vi "DMM Measurement.vi"() -> ()   [LabVIEW 2021]
doc: "This example acquires a single measurement from a National Instruments DMM. Select the measurement function and range. Specify the resolution in digits of precision. The measured value will be displayed in the Measurement indicator. The Boolean indicator will indicate if the measured value is out of range."
uses:
  <instrlib>/niDMM/nidmm.llb/niDMM Configure Measurement Digits.vi
  <instrlib>/niDMM/nidmm.llb/niDMM Function.ctl
  <instrlib>/niDMM/nidmm.llb/niDMM Resolution in Digits.ctl
panel:
  out "error out":errorcluster
  in  "error in":errorcluster caption="error in (no error)"
  in  "Resolution in Digits":T1=5.5 items=["3 1/2"=3.5, "4 1/2"=4.5, "5 1/2"=5.5, "6 1/2"=6.5, "7 1/2"=7.5]
  out "Absolute Resolution":dbl format="%#_3p"
  in  "Measurement Type":T2
  out "Signal Out of Range":bool
  in  "Range":dbl=10.0 format="%.2f"
  in  "Device Name":refnum<k15>="Dev1"
  out "Measurement":dbl format="%.6p"
  # "For instructions select File >> VI Properties >> Documentation"
  # "Configuration"
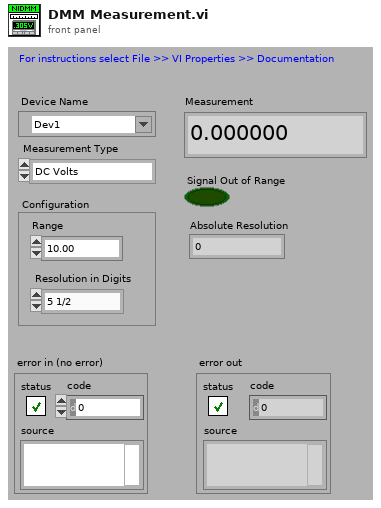
[diagram p1: front panel]
types:
  T1 = typedef "niDMM Resolution in Digits.ctl" = dbl
  T2 = typedef "niDMM Function.ctl" = enum16{"DC Volts", "AC Volts", "DC Current", "AC Current", "2-wire Resistance", "4-wire Resistance", "Diode", "Frequency", "Period", "AC Volts DC Coupled", "Capacitance", "Inductance", "Temperature"}
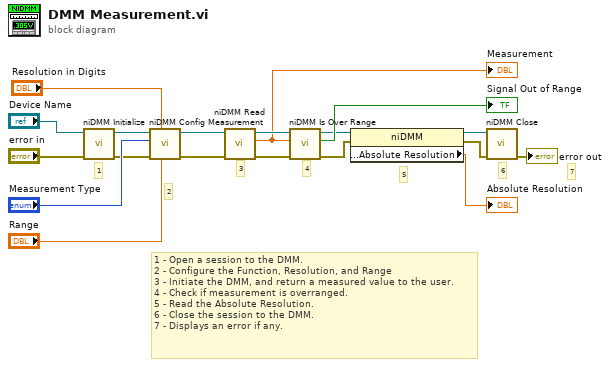
[diagram p0: block diagram]
diagram:
  # "2"
  # "1 - Open a session to the DMM.\n2 - Configure the Function, Resolution, and Range\n3 - Initiate the DMM, and return a measured value to the user.\n4 - Check if measurement is overranged.\n5 - Read the Absolute Resolution.\n6 - Close the session to the DMM.\n7 - Displays an error if any."
  # "1"
  # "7"
  # "6"
  # "5"
  # "4"
  # "3"
  n1 = call <instrlib>:"niDMM Initialize.vi"("error in (no error)"="error in", "Instrument Descriptor"="Device Name") -> ("error out"=w10:errorcluster, "instrument handle out"=w9:refnum<k15>)  [unwired: 8 in]
  n2 = call-poly <instrlib>:"niDMM Config Measurement.vi"("Range"="Range", "Resolution in Digits"="Resolution in Digits", "error in (no error)"=w10, "Function"="Measurement Type", "instrument handle"=w9) -> ("error out"=w17:errorcluster, "instrument handle out"=w16:refnum<k15>)  [unwired: 5 in]
  n3 = call <instrlib>:"niDMM Read.vi"("error in (no error)"=w17, "instrument handle"=w16) -> ("error out"=w14:errorcluster, "Measurement"=w12:dbl, "instrument handle out"=w15:refnum<k15>)  [unwired: 7 in]
  "Measurement" <- w12
  n4 = call <instrlib>:"niDMM Is Over Range.vi"("error in (no error)"=w14, "Measurement"=w12, "instrument handle"=w15) -> ("error out"=w6:errorcluster, "Over Range?"=→"Signal Out of Range":bool, "instrument handle out"=w8:refnum<k15>)  [unwired: 6 in]
  n5 = property class="niDMM"(reference=w8, error in=w6) -> (reference out=w7:refnum<k15>, error out=w5:errorcluster, "Configuration:Absolute Resolution"=→"Absolute Resolution":dbl)
  n6 = call <instrlib>:"niDMM Close.vi"("error in (no error)"=w5, "instrument handle"=w7) -> ("error out"=→"error out":errorcluster)  [unwired: 9 in]
